vi "Create and Register Sessions.vi"(8 "error in":errorcluster, 11 "Sequence Context":refnum<k7>) -> (0 "error out":errorcluster)   [LabVIEW 2020, in "Keysight 34401A DMM Measurement.lvlib"]
uses:
  Keysight 34401A DMM Measurement.lvlib
  <vilib>/MeasurementLink/MeasurementLink Session Management Client/RPC Messages/ni_measurementlink_sessionmanagement_v1_ReserveSessionsRequest.ctl
  <vilib>/MeasurementLink/MeasurementLink Session Management Client/RPC Messages/ni_measurementlink_PinMapContext.ctl
  <vilib>/MeasurementLink/MeasurementLink Discovery Client/RPC Messages/ni_measurementlink_discovery_v1_ResolveServiceRequest.ctl
  <vilib>/MeasurementLink/MeasurementLink Session Management Client/MeasurementLink Session Management Client.lvlib
  <vilib>/MeasurementLink/MeasurementLink Discovery Client/MeasurementLink Discovery Client.lvlib
  <vilib>/MeasurementLink/MeasurementLink Measurement Server/MeasurementLink Measurement Server.lvlib
  <instrlib>/Agilent 34401/Agilent 34401.lvlib
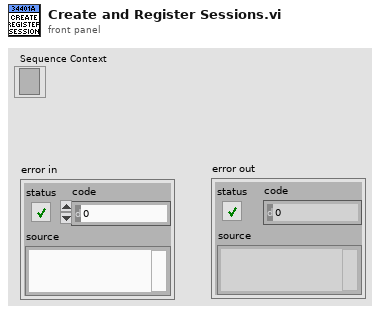
[diagram p1: front panel]
types:
  T1 = typedef "MeasurementLink Discovery Client.lvlib/ni_measurementlink_discovery_v1_ResolveServiceRequest.ctl" = cluster{"provided_interface":string, "service_class":string}
  T2 = typedef "MeasurementLink Session Management Client.lvlib/ni_measurementlink_sessionmanagement_v1_ReserveSessionsRequest.ctl" = cluster{"pin_map_context":T3, "pin_or_relay_names":string[], "instrument_type_id":string, "timeout_in_milliseconds":i32}
  T3 = typedef "MeasurementLink Session Management Client.lvlib/ni_measurementlink_PinMapContext.ctl" = cluster{"pin_map_id":string, "sites":i32[]}
  T4 = typedef "grpc-lvsupport-release.lvlib/grpcId.ctl" = u64
  T5 = typedef "MeasurementLink Discovery Client.lvlib/ni_measurementlink_discovery_v1_ServiceLocation.ctl" = cluster{"location":string, "insecure_port":string, "ssl_authenticated_port":string}
  T6 = typedef "MeasurementLink Session Management Client.lvlib/ni_measurementlink_sessionmanagement_v1_ReserveSessionsResponse.ctl" = cluster{"sessions":T7[]}
  T7 = typedef "MeasurementLink Session Management Client.lvlib/ni_measurementlink_sessionmanagement_v1_SessionInformation.ctl" = cluster{"session":T8, "resource_name":string, "channel_list":string, "instrument_type_id":string, "session_exists":bool, "channel_mappings":T9[]}
  T8 = typedef "MeasurementLink Session Management Client.lvlib/nidevice_grpc_Session.ctl" = cluster{"name":string}
  T9 = typedef "MeasurementLink Session Management Client.lvlib/ni_measurementlink_sessionmanagement_v1_ChannelMapping.ctl" = cluster{"pin_or_relay_name":string, "site":i32, "channel":string}
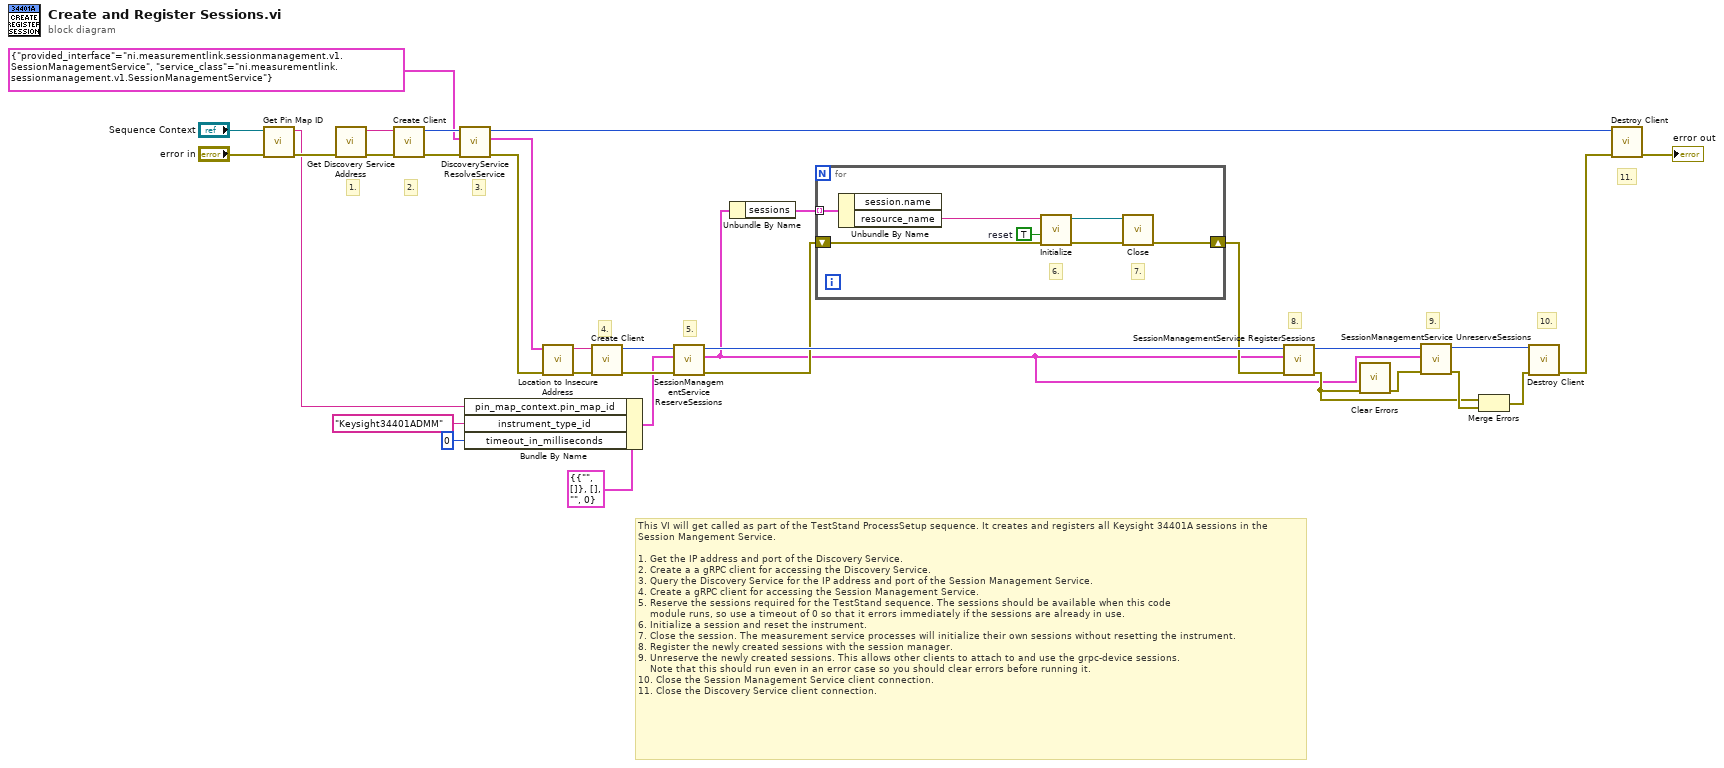
[diagram p0: block diagram]
diagram:
  # "11."
  # "10."
  # "9."
  # "8."
  # "5."
  # "4."
  # "3."
  # "2."
  # "1."
  # "This VI will get called as part of the TestStand ProcessSetup sequence. It creates and registers all Keysight 34401A sessions in the\nSession Mangement Service.\n\n1. Get the IP address and port of the Discovery Service.\n2. Create a a gRPC client for accessing the Discovery Service.\n3. Query the Discovery Service for the IP address and port of the Session Management Service.\n4. Create a gRPC client for accessing the Session Management Service.\n5. Reserve the sessions required for the TestStand sequence. The sessions should be available when this code\n    module runs, so use a timeout of 0 so that it errors immediately if the sessions are already in use.  \n6. Initialize a session and reset the instrument.\n7. Close the session. The measurement service processes will initialize their own sessions without resetting the instrument.\n8. Register the newly created sessions with the session manager.\n9. Unreserve the newly created sessions. This allows other clients to attach to and use the grpc-device sessions. \n    Note that this should run even in an error case so you should clear errors before running it.\n10. Close the Session Management Service client connection.\n11. Close the Discovery Service client connection."
  n1 = call "Get Pin Map ID.vi"("error in"="error in", "Sequence Context"="Sequence Context") -> ("error out"=w3:errorcluster, "pin_map_id"=w1:string)  [unwired: 8 in]
  n2 = call <vilib>:"Get Discovery Service Address.vi"("error in"=w3) -> ("error out"=w14:errorcluster, "address"=w13:string)  [unwired: 9 in]
  n3 = call <vilib>:"Create Client.vi"("error in"=w14, "address"=w13) -> ("error out"=w28:errorcluster, "gRPC ID Out"=w29:T4)  [unwired: 8 in]
  n4 = call <vilib>:"DiscoveryService ResolveService.vi"("error in"=w28, "Request Data"=T1 {"provided_interface"="ni.measurementlink.sessionmanagement.v1.SessionManagementService", "service_class"="ni.measurementlink.sessionmanagement.v1.SessionManagementService"}, "gRPC ID"=w29) -> ("error out"=w27:errorcluster, "Response Data"=w12:T5, "gRPC ID out"=w17:T4)  [unwired: 6 in]
  n5 = Bundle By Name(cluster=T2 {"pin_map_context"={"pin_map_id"="", "sites"=[]}, "pin_or_relay_names"=[], "instrument_type_id"="", "timeout_in_milliseconds"=0} ("Request Data"), "pin_map_context.pin_map_id"=w1, "instrument_type_id"="Keysight34401ADMM", "timeout_in_milliseconds"=0) -> (w23:T2)
  n6 = call "Location to Insecure Address.vi"("Response Data"=w12) -> ("String"=w11:string)  [unwired: 10 in]
  n7 = call <vilib>:"Create Client.vi"("error in"=w27, "address"=w11) -> ("error out"=w31:errorcluster, "gRPC ID Out"=w32:T4)  [unwired: 8 in]
  n8 = call <vilib>:"SessionManagementService ReserveSessions.vi"("error in"=w31, "Request Data"=w23, "gRPC ID"=w32) -> ("error out"=w16:errorcluster, "Response Data"=w6:T6, "gRPC ID out"=w30:T4)  [unwired: 6 in]
  n9 = Unbundle By Name(w6) -> ("sessions"=w19:T7[])
  n10 = for {
    tunnel: w19 -> [w39] mode=indexing
    shift-right: [w33] -> w22
    shift-left: w16 -> [w38]
    w36 = TRUE  # reset
    # "7."
    # "6."
    n11 = Unbundle By Name(w39) -> ("resource_name"=w37:string)  [unwired: 1 out]
    n12 = call <instrlib>:"Initialize.vi"("error in (no error)"=w38, "Reset (True)"=w36, "VISA resource name"=w37) -> ("error out"=w35:errorcluster, "VISA resource name out"=w34:refnum<visa-resource-name>)  [unwired: 7 in]
    n13 = call <instrlib>:"Close.vi"("error in (no error)"=w35, "VISA resource name"=w34) -> ("error out"=w33:errorcluster)  [unwired: 9 in]
  }
  n14 = call <vilib>:"SessionManagementService RegisterSessions.vi"("error in"=w22, "Request Data"=w6, "gRPC ID"=w30) -> ("error out"=w7:errorcluster, "gRPC ID out"=w21:T4)  [unwired: 6 in, 1 out]
  n15 = call <vilib>:"Clear Errors.vi"("error in (no error)"=w7) -> ("error out"=w10:errorcluster)  [unwired: 5 in, 1 out]
  n16 = call <vilib>:"SessionManagementService UnreserveSessions.vi"("error in"=w10, "Request Data"=w6, "gRPC ID"=w21) -> ("error out"=w9:errorcluster, "gRPC ID out"=w20:T4)  [unwired: 6 in, 1 out]
  n17 = Merge Errors(w7, w9) -> (w8:errorcluster)
  n18 = call <vilib>:"Destroy Client.vi"("error in"=w8, "gRPC ID"=w20) -> ("error out"=w26:errorcluster)  [unwired: 9 in]
  n19 = call <vilib>:"Destroy Client.vi"("error in"=w26, "gRPC ID"=w17) -> ("error out"=→"error out":errorcluster)  [unwired: 9 in]
